vi "Load Replay Samples.vi"(11 "Replay Helper Loop In":T1={"Timeout"=-1, "Run ID"="", "Replay Array Elements"=[], "User Events Metadata"=[]}) -> (3 "Replay Helper Loop Out":T1={"Timeout"=-1, "Run ID"="", "Replay Array Elements"=[], "User Events Metadata"=[]})   [LabVIEW 2026, in "Replay.lvlib"]
uses:
  Replay.lvlib
  Replay Helper Loop.ctl
  User Events Metadata.ctl
  51ae6a63-6c69-4fc5-bd9a-224650780877.vi
  <vilib>/JDP Science/JSONtext/JSON text to Variant.vi
  <vilib>/JDP Science/JSONtext/LVClass Serializer/JSONtext LVClass Serializer.lvclass
  Launcher/Launcher.lvlib
panel:
  out "error out":errorcluster
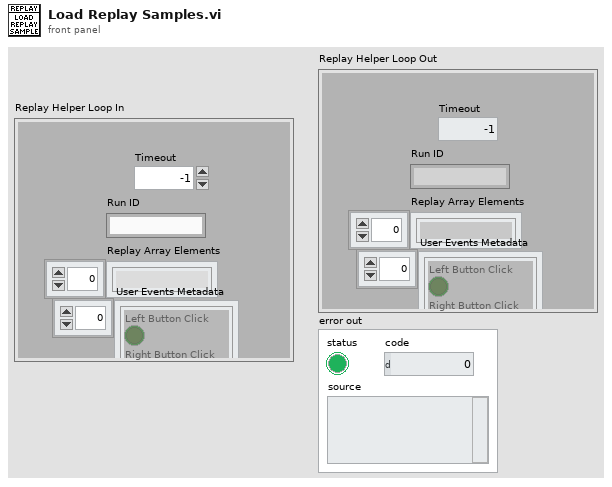
[diagram p1: front panel]
types:
  T1 = typedef "Replay.lvlib/Replay Helper Loop.ctl" = cluster{"Timeout":i32, "Run ID":string, "Replay Array Elements":string[], "User Events Metadata":T2[]}
  T2 = typedef "User Events Metadata.ctl" = cluster{"Cursor Position X":i32, "Cursor Position Y":i32, "Left Button Click":bool, "Right Button Click":bool, "Frame Number":u32}
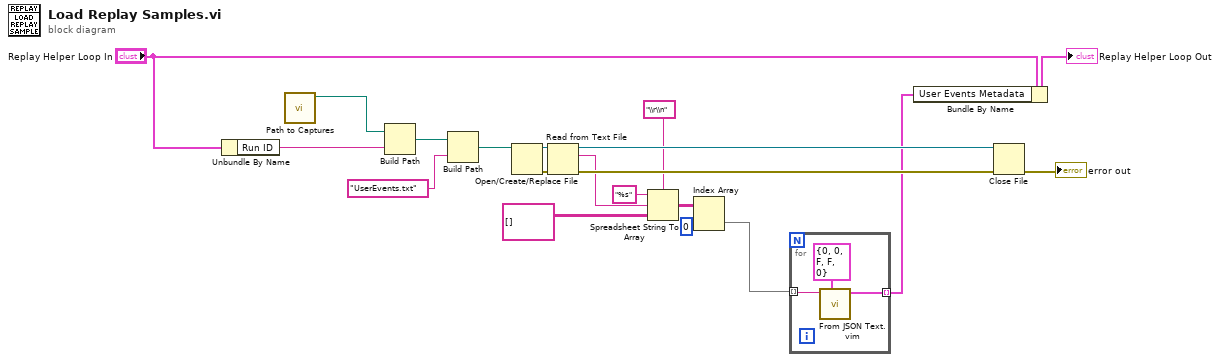
[diagram p0: block diagram]
diagram:
  n1 = Unbundle By Name("Replay Helper Loop In") -> ("Run ID"=w19:string)
  n2 = call "Path to Captures.vi"() -> ("Captures"=w20:path)  [unwired: 11 in]
  n3 = Build Path(base path=w20, name or relative path=w19) -> (appended path=w17:path)
  n4 = Build Path(base path=w17, name or relative path="UserEvents.txt" ("Run ID")) -> (appended path=w16:path)
  n5 = Open/Create/Replace File(file path (use dialog)=w16) -> (refnum out=w13:refnum<file>, error out=w15:errorcluster)  [unwired: 5 in, 1 out]
  n6 = Read from Text File(file (use dialog)=w13, error in=w15) -> (refnum out=w12:refnum<file>, text=w9:string, error out=w14:errorcluster)  [unwired: 2 in, 1 out]
  n7 = Spreadsheet String To Array(delimiter (Tab)="\\r\\n", format string="%s", spreadsheet string=w9, array type (2D Dbl)=string[][] [] ("text")) -> (array=w6:string[][])
  n8 = Index Array(array=w6, index (col)=0 ("disabled index (col)")) -> (element=w4:string[])  [unwired: 1 in]
  n9 = for {
    tunnel: w4 -> [w23] mode=indexing
    tunnel: [w21] -> w2 mode=indexing
    n10 = call "From JSON Text.vim"("Data Type and Default Value"=T2 {"Cursor Position X"=0, "Cursor Position Y"=0, "Left Button Click"=FALSE, "Right Button Click"=FALSE, "Frame Number"=0} ("User Events Metadata"), "JSON"=w23) -> ("Data out"=w21:T2)  [unwired: 8 in, 1 out]
  }
  n11 = Bundle By Name(cluster="Replay Helper Loop In", "User Events Metadata"=w2) -> (→"Replay Helper Loop Out":T1)
  n12 = Close File(refnum=w12, error in=w14) -> (error out=→"error out":errorcluster)  [unwired: 1 out]
